vi "Enable Signal Display.vi"(8 "error in (no error)":errorcluster, 9 "Enable Signal Display (T: Enable)":bool=TRUE, 10 "Signal Name (0: Channel 1)":i32(ring) items=["Channel 1", "Channel 2", "Channel 3", "Channel 4", "Function", "Waveform Memory 1", "Waveform Memory 2", "Serial Bus 1", "Serial Bus 2", "Digital Bus Low", "Digital Bus High", "Digital Bus 1", "Digital Bus 2", "D0", "D1", "D2", "D3", "D4", "D5", "D6", "D7", "D8", "D9", "D10", "D11", "D12", "D13", "D14", "D15", "External", "Line", "Waveform Generator", "Function 1", "Function 2", "Function 3", "Function 4", "Math 1", "Math 2", "Math 3", "Math 4", "Math", "FFT", "Analog Bus", "Pod 1", "Pod 2"], 11 "VISA resource name":refnum<visa-resource-name>) -> (0 "error out":errorcluster, 3 "VISA resource name out":refnum<visa-resource-name>)   [LabVIEW 2015, in "Agilent 2000 3000 X-Series.lvlib"]
doc: "Configures the front panel display of signal."
uses:
  Agilent 2000 3000 X-Series.lvlib
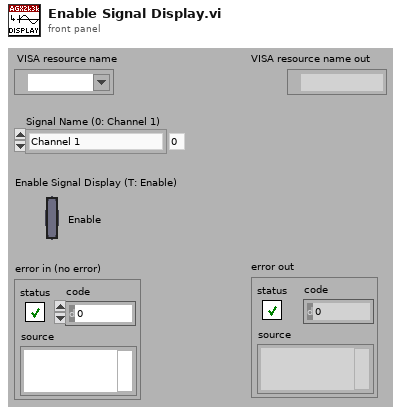
[diagram p1: front panel]
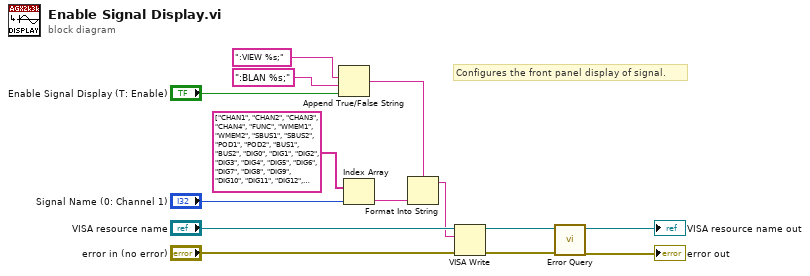
[diagram p0: block diagram]
diagram:
  # "Configures the front panel display of signal."
  n1 = Append True/False String(1:"Enable Signal Display (T: Enable)", 2:":BLAN %s;", 3:":VIEW %s;") -> (0:w5:string)  [unwired: 1 out]
  n2 = Index Array(array=string[] ["CHAN1", "CHAN2", "CHAN3", "CHAN4", "FUNC", "WMEM1", "WMEM2", "SBUS1", "SBUS2", "POD1", "POD2", "BUS1", "BUS2", "DIG0", "DIG1", "DIG2", "DIG3", "DIG4", "DIG5", "DIG6", "DIG7", "DIG8", "DIG9", "DIG10", "DIG11", "DIG12", "DIG13", "DIG14", "DIG15", "EXT", "LINE", "WGEN", "FUNC1", "FUNC2", "FUNC3", "FUNC4", "MATH1", "MATH2", "MATH3", "MATH4", "MATH", "FFT", "ABUS", "POD1", "POD2"], index="Signal Name (0: Channel 1)") -> (element=w2:string)
  n3 = Format Into String(format string=w5, w2) -> (resulting string=w4:string)  [unwired: 2 in, 1 out]
  n4 = VISA Write(VISA resource name="VISA resource name", write buffer=w4, error in (no error)="error in (no error)") -> (VISA resource name out=w12:refnum<visa-resource-name>, error out=w11:errorcluster)  [unwired: 1 out]
  n5 = call "Error Query.vi"("error in (no error)"=w11, "VISA resource name"=w12) -> ("error out"=→"error out":errorcluster, "VISA resource name out"=→"VISA resource name out":refnum<visa-resource-name>)  [unwired: 8 out]
